vi "BioMapHeaderWriter.vi"(8 "error in":errorcluster, 9 "Pixel Dimension":T1={"Dimension 1"=1.0, "Dimension 2"=1.0, "Dimension 3"=1.0, "Dimension 4"=1.0, "Dimension 5"=0.0, "Dimension 6"=0.0, "Dimension 7"=0.0, "Dimension 8"=0.0}, 10 "Dimensions":T2={"Dimension"=4, "SpecDepth"=0, "x dimension"=0, "y dimension"=0, "z dimension"=1}, 11 "image file path":path) -> (0 "error out":errorcluster)   [LabVIEW 2011]
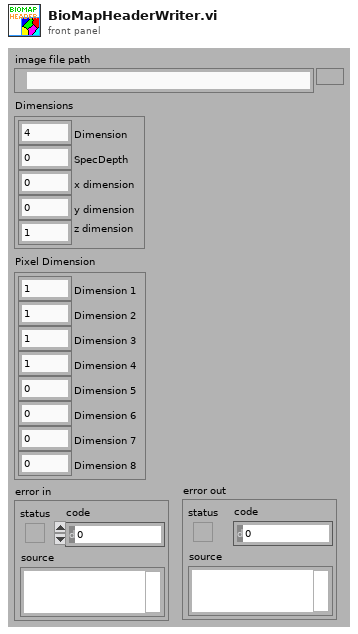
[diagram p1: front panel]
types:
  T1 = cluster{"Dimension 1":sgl, "Dimension 2":sgl, "Dimension 3":sgl, "Dimension 4":sgl, "Dimension 5":sgl, "Dimension 6":sgl, "Dimension 7":sgl, "Dimension 8":sgl}
  T2 = cluster{"Dimension":u16, "SpecDepth":u16, "x dimension":u16, "y dimension":u16, "z dimension":u16}
  T3 = enum16{"big-endian, network order", "native, host order", "little-endian"}
  T4 = enum16{"open", "replace", "create", "open or create", "replace or create", "replace or create with confirmation"}
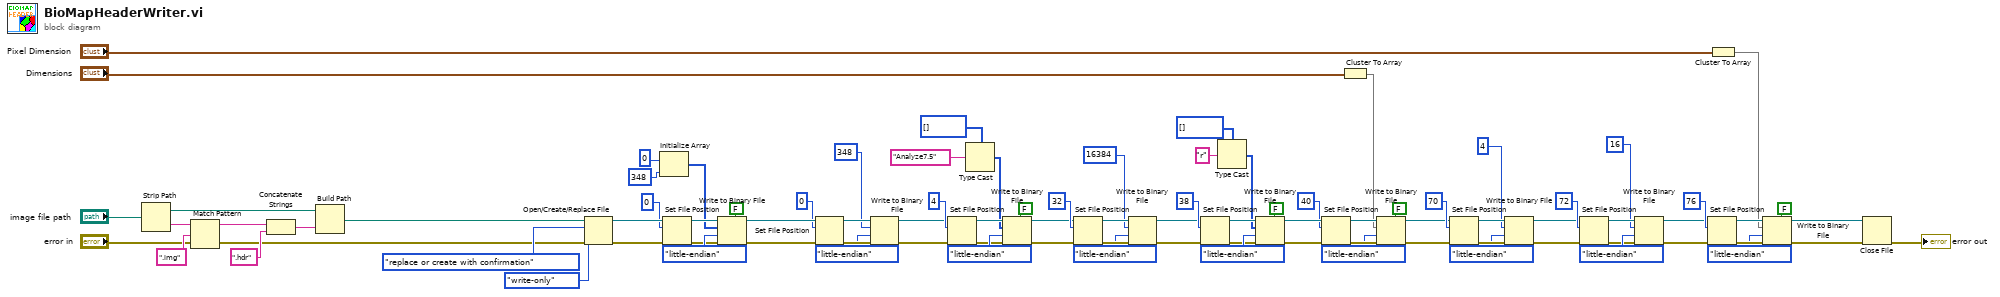
[diagram p0: block diagram]
diagram:
  n1 = Strip Path(path="image file path") -> (stripped path=w5:path, name=w9:string)
  n2 = Match Pattern(string=w9, regular expression=".img" ("string")) -> (before substring=w8:string)  [unwired: 1 in, 3 out]
  n3 = Concatenate Strings(w8, ".hdr" ("string")) -> (w6:string)
  n4 = Build Path(base path=w5, name or relative path=w6) -> (appended path=w4:path)
  n5 = Open/Create/Replace File(file path (use dialog)=w4, error in="error in", operation (0:open)=T4."replace or create with confirmation", access (0:read/write)=enum16{"read/write", "read-only", "write-only"}."write-only") -> (refnum out=w85:refnum<file>, error out=w83:errorcluster)  [unwired: 2 in, 1 out]
  n6 = Initialize Array(u8 0, 348 ("dimension size")) -> (w72:u8[])
  n7 = Set File Position(offset (in bytes) (0)=i64 0, refnum=w85, error in=w83) -> (refnum out=w84:refnum<file>, error out=w82:errorcluster)  [unwired: 1 in]
  n8 = Write to Binary File(file (use dialog)=w84, data=w72, error in=w82, 5:FALSE ("prepend array or string size? (T)"), 9:T3."little-endian" ("byte order (0:big-endian, network order)")) -> (refnum out=w76:refnum<file>, error out=w77:errorcluster)  [unwired: 1 in, 1 out]
  n9 = Set File Position(offset (in bytes) (0)=i64 0, refnum=w76, error in=w77) -> (refnum out=w79:refnum<file>, error out=w80:errorcluster)  [unwired: 1 in]
  n10 = Write to Binary File(file (use dialog)=w79, data=348, error in=w80, 9:T3."little-endian" ("byte order (0:big-endian, network order)")) -> (refnum out=w66:refnum<file>, error out=w65:errorcluster)  [unwired: 2 in, 1 out]
  n11 = Set File Position(offset (in bytes) (0)=i64 4, refnum=w66, error in=w65) -> (refnum out=w68:refnum<file>, error out=w67:errorcluster)  [unwired: 1 in]
  n12 = Type Cast(type=u8[] [], x="Analyze7.5") -> (*(type *) &x=w42:u8[])
  n13 = Write to Binary File(file (use dialog)=w68, data=w42, error in=w67, 5:FALSE ("prepend array or string size? (T)"), 9:T3."little-endian" ("byte order (0:big-endian, network order)")) -> (refnum out=w19:refnum<file>, error out=w20:errorcluster)  [unwired: 1 in, 1 out]
  n14 = Set File Position(offset (in bytes) (0)=i64 32, refnum=w19, error in=w20) -> (refnum out=w63:refnum<file>, error out=w64:errorcluster)  [unwired: 1 in]
  n15 = Write to Binary File(file (use dialog)=w63, data=16384, error in=w64, 9:T3."little-endian" ("byte order (0:big-endian, network order)")) -> (refnum out=w22:refnum<file>, error out=w21:errorcluster)  [unwired: 2 in, 1 out]
  n16 = Set File Position(offset (in bytes) (0)=i64 38, refnum=w22, error in=w21) -> (refnum out=w58:refnum<file>, error out=w57:errorcluster)  [unwired: 1 in]
  n17 = Type Cast(type=u8[] [], x="r") -> (*(type *) &x=w40:u8[])
  n18 = Write to Binary File(file (use dialog)=w58, data=w40, error in=w57, 5:FALSE ("prepend array or string size? (T)"), 9:T3."little-endian" ("byte order (0:big-endian, network order)")) -> (refnum out=w31:refnum<file>, error out=w38:errorcluster)  [unwired: 1 in, 1 out]
  n19 = Set File Position(offset (in bytes) (0)=i64 40, refnum=w31, error in=w38) -> (refnum out=w54:refnum<file>, error out=w53:errorcluster)  [unwired: 1 in]
  n20 = Cluster To Array(cluster="Dimensions") -> (array=w29:u16[])
  n21 = Write to Binary File(file (use dialog)=w54, data=w29, error in=w53, 5:FALSE ("prepend array or string size? (T)"), 9:T3."little-endian" ("byte order (0:big-endian, network order)")) -> (refnum out=w32:refnum<file>, error out=w37:errorcluster)  [unwired: 1 in, 1 out]
  n22 = Set File Position(offset (in bytes) (0)=i64 70, refnum=w32, error in=w37) -> (refnum out=w55:refnum<file>, error out=w56:errorcluster)  [unwired: 1 in]
  n23 = Write to Binary File(file (use dialog)=w55, data=i16 4, error in=w56, 9:T3."little-endian" ("byte order (0:big-endian, network order)")) -> (refnum out=w33:refnum<file>, error out=w36:errorcluster)  [unwired: 2 in, 1 out]
  n24 = Set File Position(offset (in bytes) (0)=i64 72, refnum=w33, error in=w36) -> (refnum out=w45:refnum<file>, error out=w44:errorcluster)  [unwired: 1 in]
  n25 = Write to Binary File(file (use dialog)=w45, data=i16 16, error in=w44, 9:T3."little-endian" ("byte order (0:big-endian, network order)")) -> (refnum out=w34:refnum<file>, error out=w35:errorcluster)  [unwired: 2 in, 1 out]
  n26 = Set File Position(offset (in bytes) (0)=i64 76, refnum=w34, error in=w35) -> (refnum out=w50:refnum<file>, error out=w51:errorcluster)  [unwired: 1 in]
  n27 = Cluster To Array(cluster="Pixel Dimension") -> (array=w25:sgl[])
  n28 = Write to Binary File(file (use dialog)=w50, data=w25, error in=w51, 5:FALSE ("prepend array or string size? (T)"), 9:T3."little-endian" ("byte order (0:big-endian, network order)")) -> (refnum out=w23:refnum<file>, error out=w24:errorcluster)  [unwired: 1 in, 1 out]
  n29 = Close File(refnum=w23, error in=w24) -> (error out=→"error out":errorcluster)  [unwired: 1 out]
